vi "VFH-View-R140.vi"() -> ()   [LabVIEW 2020, in "VFH-VNA_File_Handler.lvlib"]
uses:
  VFH-VNA_File_Handler.lvlib
panel:
  out "Raw 2":T1(graph)
  in  "file path (dialog if empty) 2":path=path "C:/projects/UNI/VNA/MiniVNA/20240625-162312-Vann/Vann.txt"
  out "Raw":T1(graph)
  in  "file path (dialog if empty)":path=path "C:/projects/UNI/VNA/MiniVNA/20240625-162312-Vann/Vann.txt"
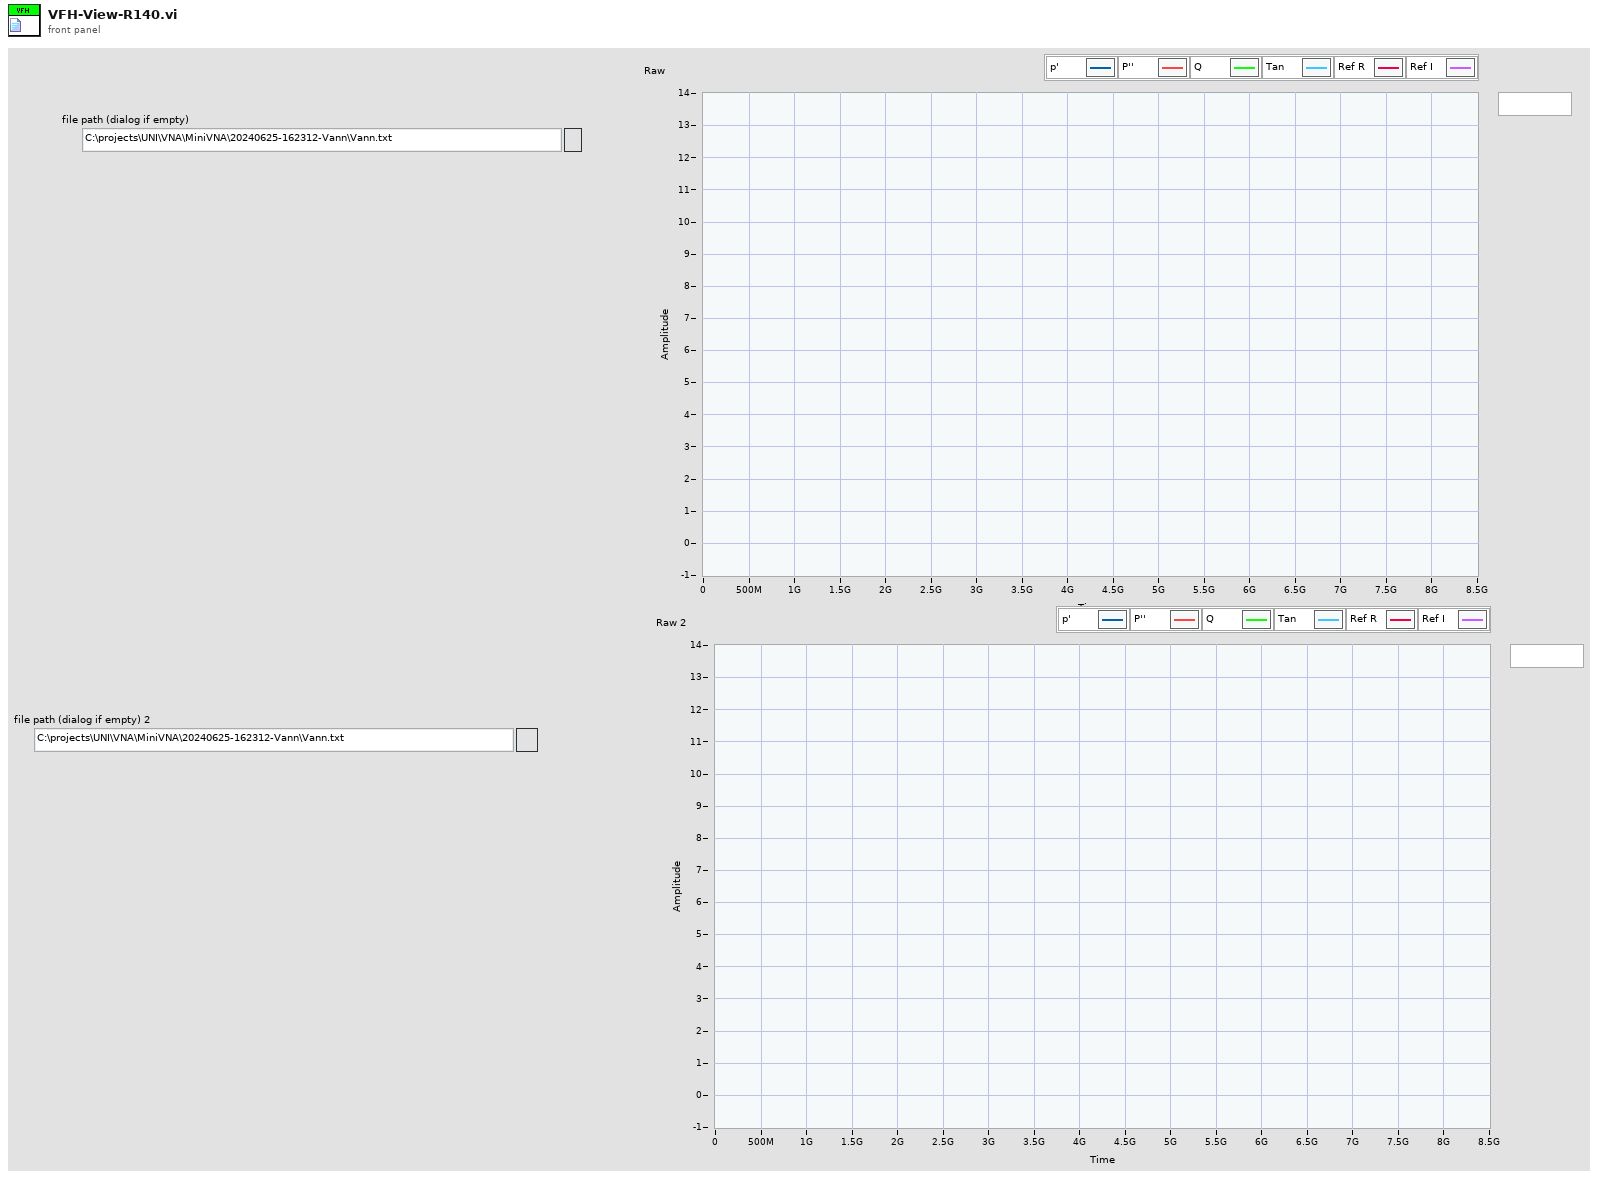
[diagram p1: front panel]
types:
  T1 = cluster{"Frequency":dbl[], "Reflection R":dbl[]}[]
  T2 = typedef "VFH-VNA_File_Handler.lvlib/VFH-file_cluster-R140.ctl" = cluster{"Frequency":dbl[], "Permativity'":dbl[], "Permativity''":dbl[], "Q [S/m]":dbl[], "Tan":dbl[], "Reflection R":dbl[], "Reflection I":dbl[]}
  T3 = cluster{"Frequency":dbl[], "Permativity''":dbl[]}
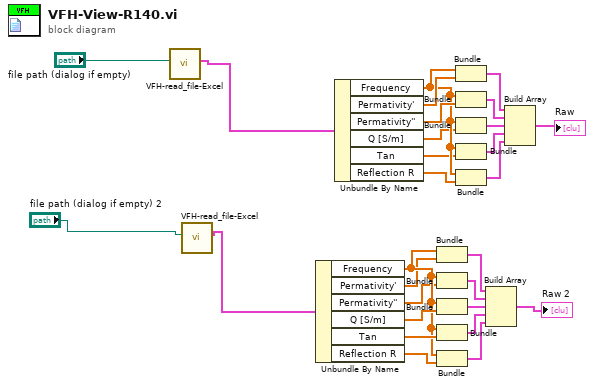
[diagram p0: block diagram]
diagram:
  n1 = call "VFH-read_file-Excel.vi"("file path (dialog if empty)"="file path (dialog if empty)") -> ("output cluster"=w3:T2)  [unwired: 9 in, 1 out]
  n2 = call "VFH-read_file-Excel.vi"("file path (dialog if empty)"="file path (dialog if empty) 2") -> ("output cluster"=w1:T2)  [unwired: 9 in, 1 out]
  n3 = Unbundle By Name(w1) -> ("Frequency"=w8:dbl[], "Permativity'"=w6:dbl[], "Permativity''"=w7:dbl[], "Q [S/m]"=w9:dbl[], "Tan"=w10:dbl[], "Reflection R"=w11:dbl[])
  n4 = Unbundle By Name(w3) -> ("Frequency"=w26:dbl[], "Permativity'"=w28:dbl[], "Permativity''"=w27:dbl[], "Q [S/m]"=w25:dbl[], "Tan"=w24:dbl[], "Reflection R"=w23:dbl[])
  n5 = Bundle("Frequency"=w8, "Permativity'"=w6) -> (w12:cluster{"Frequency":dbl[], "Permativity'":dbl[]})  [unwired: 1 in]
  n6 = Bundle("Frequency"=w8, "Permativity''"=w7) -> (w13:T3)  [unwired: 1 in]
  n7 = Bundle("Frequency"=w8, "Q [S/m]"=w9) -> (w14:cluster{"Frequency":dbl[], "Q [S/m]":dbl[]})  [unwired: 1 in]
  n8 = Bundle("Frequency"=w8, "Tan"=w10) -> (w15:cluster{"Frequency":dbl[], "Tan":dbl[]})  [unwired: 1 in]
  n9 = Bundle("Frequency"=w8, "Reflection R"=w11) -> (w16:cluster{"Frequency":dbl[], "Reflection R":dbl[]})  [unwired: 1 in]
  n10 = Bundle("Frequency"=w26, "Permativity'"=w28) -> (w22:cluster{"Frequency":dbl[], "Permativity'":dbl[]})  [unwired: 1 in]
  n11 = Bundle("Frequency"=w26, "Permativity''"=w27) -> (w21:T3)  [unwired: 1 in]
  n12 = Bundle("Frequency"=w26, "Q [S/m]"=w25) -> (w20:cluster{"Frequency":dbl[], "Q [S/m]":dbl[]})  [unwired: 1 in]
  n13 = Bundle("Frequency"=w26, "Tan"=w24) -> (w19:cluster{"Frequency":dbl[], "Tan":dbl[]})  [unwired: 1 in]
  n14 = Bundle("Frequency"=w26, "Reflection R"=w23) -> (w18:cluster{"Frequency":dbl[], "Reflection R":dbl[]})  [unwired: 1 in]
  n15 = Build Array(w12, w13, w14, w15, w16) -> (→"Raw 2":T1)
  n16 = Build Array(w22, w21, w20, w19, w18) -> (→"Raw":T1)
